vi "Clear.vi"(8 "error in (no error)":errorcluster, 10 "Network":string, 11 "MicronCLI in":refnum<class "MicronCLI.lvclass">) -> (0 "error out":errorcluster, 3 "MicronCLI out":refnum<class "MicronCLI.lvclass">)   [LabVIEW 2019, in "MicronCLI.lvclass"]
uses:
  MicronCLI.lvclass
  MicronCLI.lvclass/MicronCLI.ctl
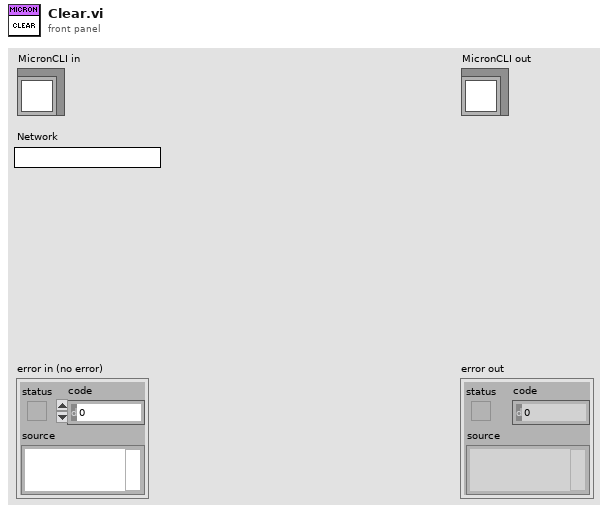
[diagram p1: front panel]
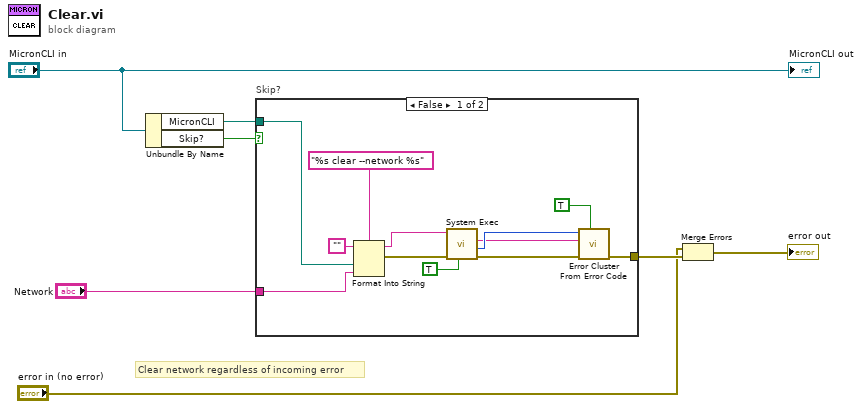
[diagram p0: block diagram]
diagram:
  # "Clear network regardless of incoming error"
  n1 = Unbundle By Name("MicronCLI in") -> ("MicronCLI"=w4:path, "Skip?"=w3:bool)
  n2 = case "Skip?" shown="False" w3 {
    tunnel: w4 -> [w16 _]
    tunnel: [w12 _] -> w7
    tunnel: "Network" -> [w8 _]
    frame False {
      n3 = Format Into String(format string="%s clear --network %s", initial string="", w16, w8) -> (resulting string=w14:string, error out=w18:errorcluster)  [unwired: 1 in]
      n4 = call <vilib>:"System Exec.vi"("run minimized? (F)"=TRUE, "error in (no error)"=w18, "command line"=w14) -> ("error out"=w19:errorcluster, "return code"=w11:i32, "standard error"=w10:string)  [unwired: 5 in, 1 out]
      n5 = call <vilib>:"Error Cluster From Error Code.vi"("show call chain? (False)"=TRUE, "error in (no error)"=w19, "error message (\"\")"=w10, "error code (0)"=w11) -> ("error out"=w12:errorcluster)  [unwired: 5 in]
    }
    frame True {
    }
  }
  n6 = Merge Errors("error in (no error)", w7) -> (→"error out":errorcluster)
  "MicronCLI out" <- "MicronCLI in"
